vi "S2C_FORNAX_Poly_VolumeBarsCommand.vi"(8 "Error In":errorcluster, 10 "VolumeBarsCommand":T2={"Partition"="Default", "Message"="VolumeBarsCommand", "M_VolumeBarsCommand"=0} {"M_VolumeBarsCommand" items=["VOLUME_COMMAND_NO_CHANGE", "VOLUME_COMMAND_INCREASE", "VOLUME_COMMAND_DECREASE", "VOLUME_COMMAND_SET_TO_ZERO", "VOLUME_COMMAND_CLOSE_OVERLAY"]}, 11 "Settings":T3={"Driver"="Fornax", "Command"="VolumeBarsCommand", "Return"="ErrorStatus", "Parameters"="", "Timeout"=10.0}) -> (0 "Error Out":errorcluster, 3 "Response":string)   [LabVIEW 2015]
uses:
  Typedefs/VolumeCommand.ctl
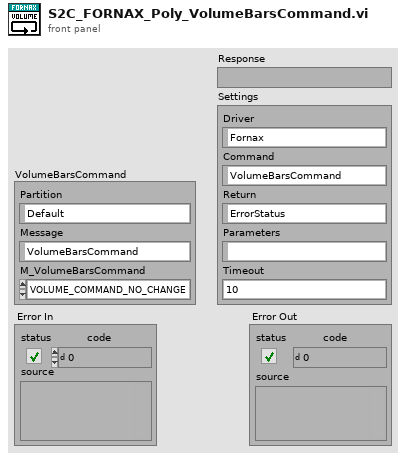
[diagram p1: front panel]
types:
  T1 = typedef "VolumeCommand.ctl" = i16
  T2 = cluster{"Partition":string, "Message":string, "M_VolumeBarsCommand":T1}
  T3 = cluster{"Driver":string, "Command":string, "Return":string, "Parameters":string, "Timeout":dbl}
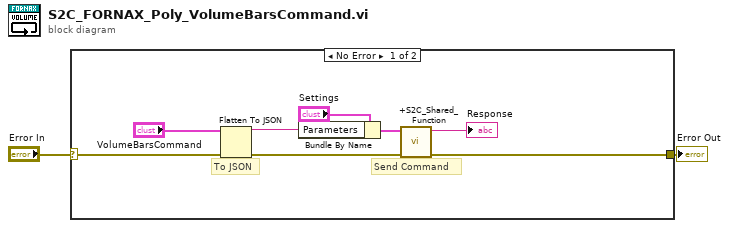
[diagram p0: block diagram]
diagram:
  n1 = case shown="No Error" "Error In" {
    selector: "Error In" -> [w6 w11]
    tunnel: [w5 w11] -> w1
    frame No Error {
      # "To JSON"
      # "Send Command"
      n2 = Flatten To JSON(anything="VolumeBarsCommand", error in (no error)=w6) -> (JSON string=w7:string, 11:w9:errorcluster)  [unwired: 1 in]
      n3 = Bundle By Name(cluster="Settings", "Parameters"=w7) -> (w10:T3)
      n4 = call "+S2C_Shared_Function.vi"("Error In"=w9, "Settings"=w10) -> ("Error Out"=w5:errorcluster, "Response"=→"Response":string)  [unwired: 8 in]
    }
    frame Error {
    }
  }
  "Error Out" <- w1
